vi "Write TDMS.vi"(0 "Queue In":refnum<queue>, 1 "TDMS File In":refnum<k34>, 2 "TDMS Group Names":T3, 3 "Elements Remaning":u32[](array[numeric]), 4 "Logging Channel Cluster":T2, 5 "FIFO Cluster":T1) -> (14 "Logging Channel Cluster":T3, 15 "TDMS Out":refnum<k34>, 16 "Elements Remaining Out":u32[](array[numeric]), 17 "Logging Channel Cluster":T2)   [LabVIEW 2017]
uses:
  Message Queue/Message Cluster.ctl
  Controls/Logging names.ctl
  Message Queue/Message Queue.lvlib
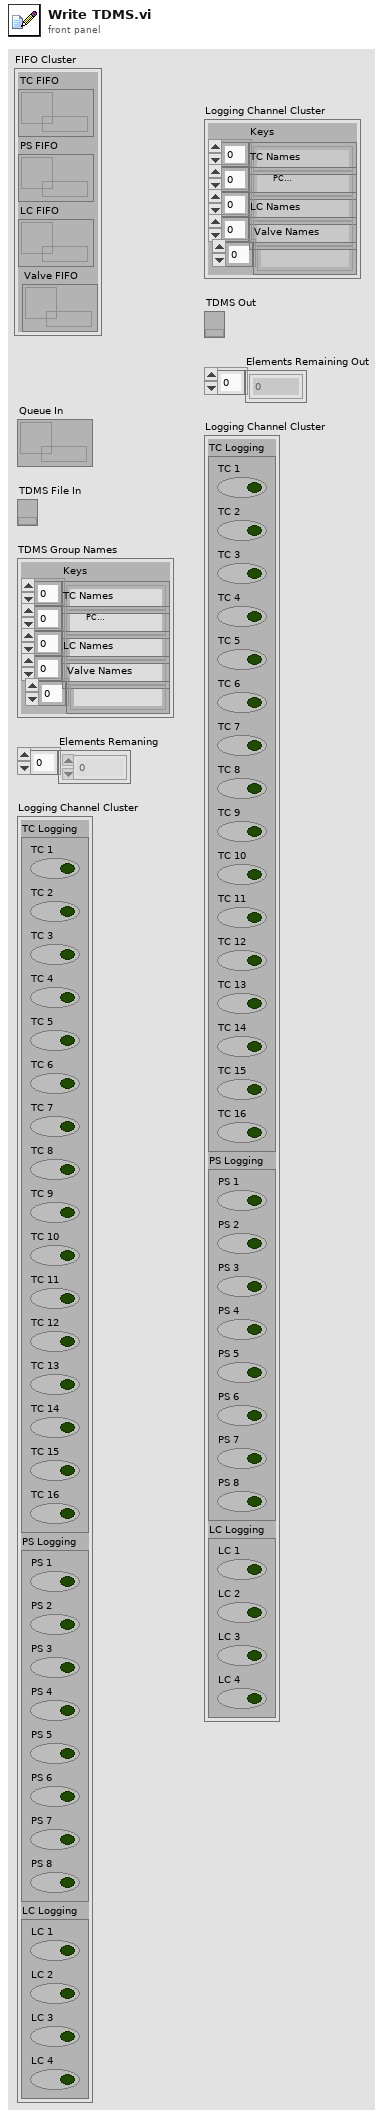
[diagram p1: front panel]
types:
  T1 = cluster{"TC FIFO":refnum<k33>, "PS FIFO":refnum<k33>, "LC FIFO":refnum<k33>, "Valve FIFO":refnum<k33>}
  T2 = cluster{"TC Logging":cluster{"TC 1":bool, "TC 2":bool, "TC 3":bool, "TC 4":bool, "TC 5":bool, "TC 6":bool, "TC 7":bool, "TC 8":bool, "TC 9":bool, "TC 10":bool, "TC 11":bool, "TC 12":bool, "TC 13":bool, "TC 14":bool, "TC 15":bool, "TC 16":bool}, "PS Logging":cluster{"PS 1":bool, "PS 2":bool, "PS 3":bool, "PS 4":bool, "PS 5":bool, "PS 6":bool, "PS 7":bool, "PS 8":bool}, "LC Logging":cluster{"LC 1":bool, "LC 2":bool, "LC 3":bool, "LC 4":bool}}
  T3 = typedef "Logging names.ctl" = cluster{"Keys":string[], "TC Names":string[], "PC Names":string[], "LC Names":string[], "Valve Names":string[]}
  T4 = cluster{"TC 1":bool, "TC 2":bool, "TC 3":bool, "TC 4":bool, "TC 5":bool, "TC 6":bool, "TC 7":bool, "TC 8":bool, "TC 9":bool, "TC 10":bool, "TC 11":bool, "TC 12":bool, "TC 13":bool, "TC 14":bool, "TC 15":bool, "TC 16":bool}
  T5 = cluster{"PS 1":bool, "PS 2":bool, "PS 3":bool, "PS 4":bool, "PS 5":bool, "PS 6":bool, "PS 7":bool, "PS 8":bool}
  T6 = cluster{"LC 1":bool, "LC 2":bool, "LC 3":bool, "LC 4":bool}
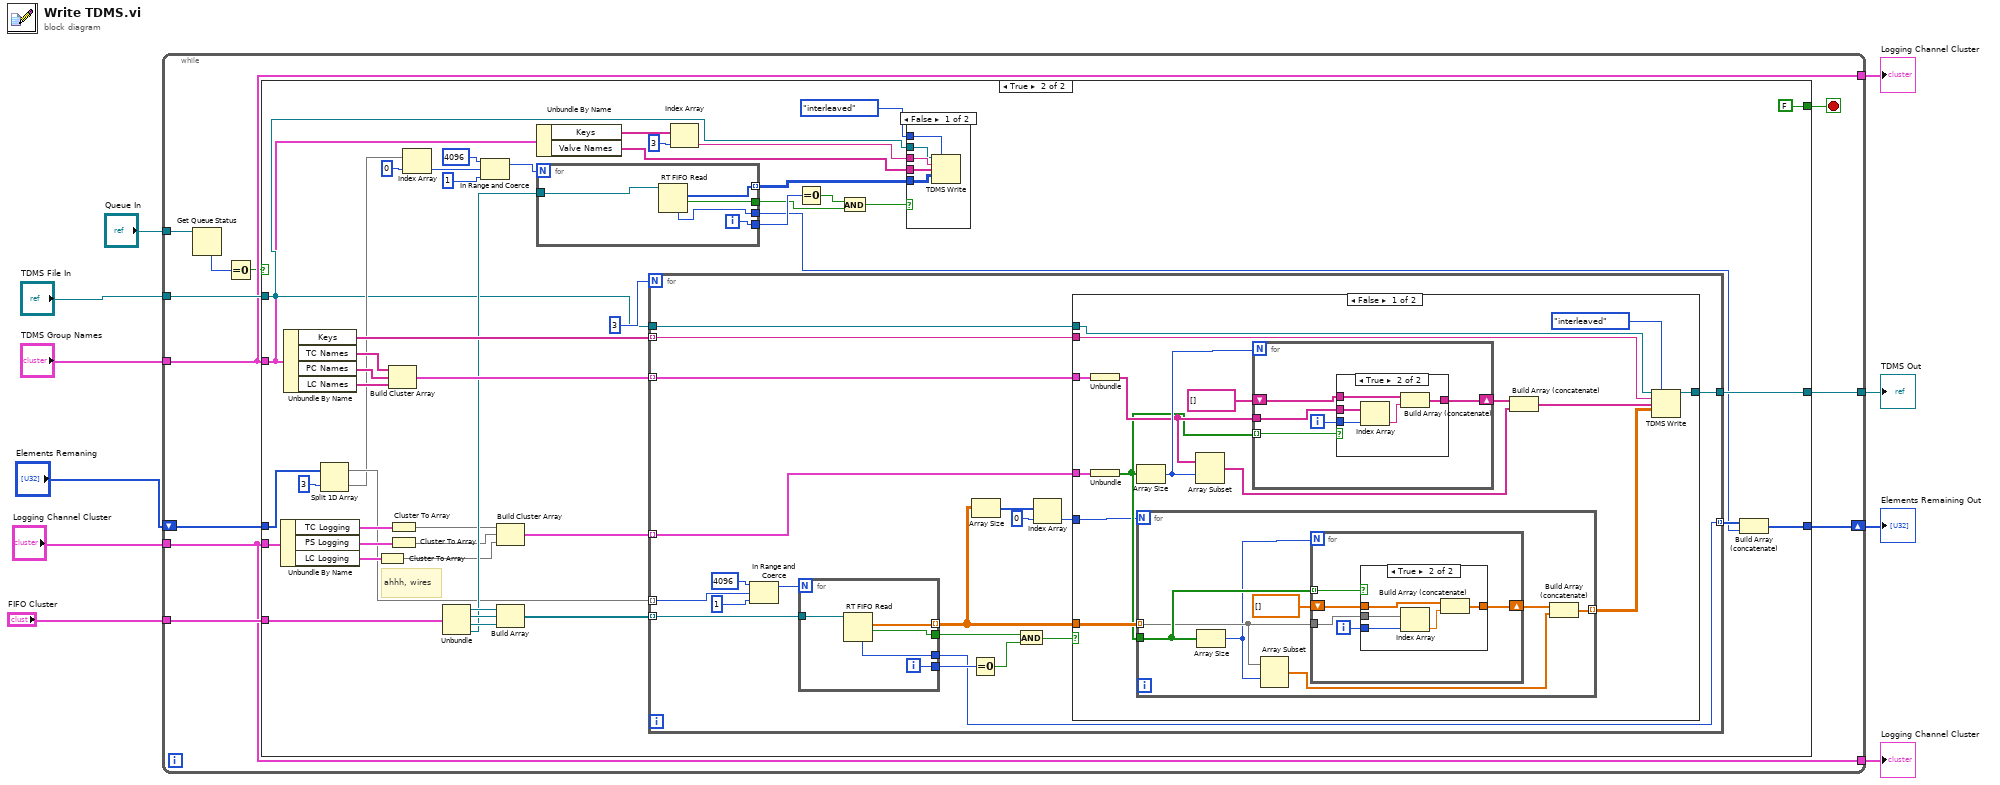
[diagram p0: block diagram]
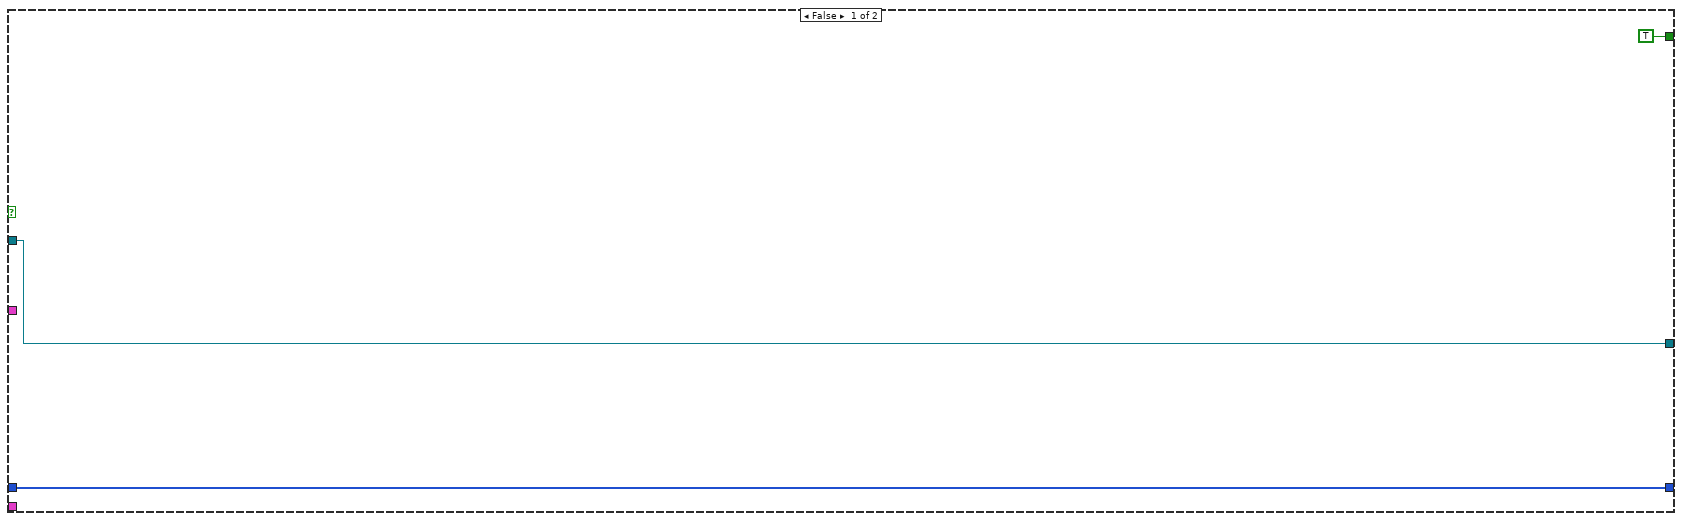
[diagram p2: hidden frame]
diagram:
  n1 = while {
    tunnel: "FIFO Cluster" -> [w17]
    tunnel: [w21] -> w2
    tunnel: "Logging Channel Cluster" -> [w15]
    tunnel: "TDMS Group Names" -> [w16]
    tunnel: "TDMS File In" -> [w18]
    shift-right: [w19] -> w5
    shift-left: "Elements Remaning" -> [w20]
    tunnel: [w15] -> w9
    tunnel: [w16] -> w8
    tunnel: "Queue In" -> [w14]
    stop <- w11 stop-if-true
    n2 = Get Queue Status(queue=w14) -> (# elements in queue=w12:i32)  [unwired: 2 in, 7 out]
    n3 = Equal To 0?(x=w12) -> (x = 0?=w13:bool)
    n4 = case shown="True" w13 {
      tunnel: [w22 w54] -> w21
      tunnel: w20 -> [w23 w41]
      tunnel: [w23 w36] -> w19
      tunnel: w18 -> [w22 w29]
      tunnel: w17 -> [_ w28]
      tunnel: w16 -> [_ w27]
      tunnel: w15 -> [_ w26]
      tunnel: [TRUE FALSE] -> w11
      frame False {
      }
      frame True {
        # "ahhh, wires"
        n5 = Unbundle By Name(w26) -> ("TC Logging"=w53:T4, "PS Logging"=w52:T5, "LC Logging"=w51:T6)
        n6 = Unbundle By Name(w27) -> ("Keys"=w61:string[], "TC Names"=w70:string[], "PC Names"=w69:string[], "LC Names"=w68:string[])
        n7 = Split 1D Array(array=w41, index=3) -> (first subarray=w39:u32[], second subarray=w38:u32[])
        n8 = Cluster To Array(cluster=w51) -> (array=w48:bool[])
        n9 = Build Cluster Array(w70, w69, w68) -> (w62:cluster{"LC Names":string[]}[])
        n10 = Cluster To Array(cluster=w53) -> (array=w50:bool[])
        n11 = Cluster To Array(cluster=w52) -> (array=w49:bool[])
        n12 = Index Array(array=w38, index=0) -> (element=w32:u32)
        n13 = Unbundle(w28) -> ("TC FIFO"=w64:refnum<k33>, "PS FIFO"=w65:refnum<k33>, "LC FIFO"=w66:refnum<k33>, "Valve FIFO"=w60:refnum<k33>)
        n14 = In Range and Coerce(upper limit=u32 4096, x=w32, lower limit=u32 1) -> (coerced(x)=w33:u32)  [unwired: 1 out]
        n15 = Build Cluster Array(w50, w49, w48) -> (w47:cluster{"LC Logging":bool[]}[])
        n16 = Build Array(w64, w65, w66) -> (w63:refnum<k33>[])
        n17 = Unbundle By Name(w27) -> ("Keys"=w59:string[], "Valve Names"=w56:string[])
        n18 = for {
          N: w33 -> [_]
          tunnel: [w74] -> w46 mode=indexing
          tunnel: w60 -> [w75]
          tunnel: [w73] -> w44
          tunnel: [w72] -> w42
          tunnel: [w71] -> w30
          i -> [w73]
          n19 = RT FIFO Read(0:w75) -> (7:w71:u32, 9:w74:i32[], 10:w72:bool)  [unwired: 3 in, 2 out]
        }
        n20 = for {
          N: 3 -> [_]
          tunnel: w63 -> [w99] mode=indexing
          tunnel: w62 -> [w95] mode=indexing
          tunnel: w61 -> [w98] mode=indexing
          tunnel: [w97] -> w54
          tunnel: w47 -> [w94] mode=indexing
          tunnel: w39 -> [w82] mode=indexing
          tunnel: [w86] -> w37 mode=indexing
          tunnel: w29 -> [w81]
          n21 = In Range and Coerce(upper limit=u32 4096, x=w82, lower limit=u32 1) -> (coerced(x)=w83:u32)  [unwired: 1 out]
          n22 = for {
            N: w83 -> [_]
            tunnel: w99 -> [w104]
            tunnel: [w103] -> w96 mode=indexing
            tunnel: [w102] -> w90
            tunnel: [w101] -> w87
            tunnel: [w100] -> w86
            i -> [w102]
            n23 = RT FIFO Read(0:w104) -> (7:w100:u32, 9:w103:sgl[], 10:w101:bool)  [unwired: 3 in, 2 out]
          }
          n24 = Equal To 0?(x=w90) -> (x = 0?=w89:bool)
          n25 = Array Size(array=w96) -> (size(s)=w91:i32[])
          n26 = And(x=w87, y=w89) -> (x .and. y?=w88:bool)
          n27 = Index Array(array=w91, index=0) -> (element=w92:i32)
          n28 = case shown="False" w88 {
            tunnel: w98 -> [w120 _]
            tunnel: [w118 w150] -> w97
            tunnel: w96 -> [w116 _]
            tunnel: w95 -> [w111 _]
            tunnel: w94 -> [w109 _]
            tunnel: w92 -> [w106 _]
            tunnel: w81 -> [w105 w150]
            frame False {
              n29 = Unbundle(w111) -> ("LC Names"=w110:string[])
              n30 = Unbundle(w109) -> ("LC Logging"=w108:bool[])
              n31 = Array Size(array=w108) -> (size(s)=w113:i32)
              n32 = for {
                N: w106 -> [_]
                tunnel: w116 -> [w125] mode=indexing
                tunnel: w108 -> [w127]
                tunnel: [w121] -> w107 mode=indexing
                n33 = Array Size(array=w127) -> (size(s)=w124:i32)
                n34 = Array Subset(array=w125, index=w124) -> (w122:sgl[])  [unwired: 1 in]
                n35 = for {
                  N: w124 -> [_]
                  tunnel: w127 -> [w131] mode=indexing
                  tunnel: w125 -> [w130]
                  shift-right: [w129] -> w123
                  shift-left: sgl[] [] -> [w128]
                  i -> [w132]
                  n36 = case shown="True" w131 {
                    tunnel: w132 -> [_ w138]
                    tunnel: w130 -> [_ w135]
                    tunnel: [w133 w137] -> w129
                    tunnel: w128 -> [w133 w134]
                    frame False {
                    }
                    frame True {
                      n37 = Index Array(array=w135, index=w138) -> (element=w136:sgl)
                      n38 = Build Array (concatenate)(w134, w136) -> (w137:sgl[])
                    }
                  }
                }
                n39 = Build Array (concatenate)(w123, w122) -> (w121:sgl[])
              }
              n40 = Array Subset(array=w110, index=w113) -> (w112:string[])  [unwired: 1 in]
              n41 = for {
                N: w113 -> [_]
                tunnel: w108 -> [w143] mode=indexing
                tunnel: w110 -> [w141]
                shift-right: [w139] -> w114
                shift-left: string[] [] -> [w140]
                i -> [w142]
                n42 = case shown="True" w143 {
                  tunnel: w142 -> [_ w148]
                  tunnel: w141 -> [_ w149]
                  tunnel: w140 -> [w144 w146]
                  tunnel: [w144 w145] -> w139
                  frame False {
                  }
                  frame True {
                    n43 = Index Array(array=w149, index=w148) -> (element=w147:string)
                    n44 = Build Array (concatenate)(w146, w147) -> (w145:string[])
                  }
                }
              }
              n45 = Build Array (concatenate)(w114, w112) -> (w117:string[])
              n46 = TDMS Write(0:w105, 1:enum16{"decimated", "interleaved"}."interleaved" ("data layout (0:decimated)"), 5:w120, 7:w117, 9:w107) -> (4:w118:refnum<k34>)  [unwired: 1 in, 3 out]
            }
            frame True {
            }
          }
        }
        n47 = Index Array(array=w59, index=3) -> (element=w57:string)
        n48 = Equal To 0?(x=w44) -> (x = 0?=w45:bool)
        n49 = And(x=w45, y=w42) -> (x .and. y?=w43:bool)
        n50 = case shown="False" w43 {
          tunnel: w46 -> [w80 _]
          tunnel: w57 -> [w79 _]
          tunnel: w29 -> [w78 _]
          tunnel: w56 -> [w77 _]
          tunnel: enum16{"decimated", "interleaved"}."interleaved" ("data layout (0:decimated)") -> [w76 _]
          frame False {
            n51 = TDMS Write(0:w78, 1:w76, 5:w79, 7:w77, 9:w80) -> ()  [unwired: 1 in, 4 out]
          }
          frame True {
          }
        }
        n52 = Build Array (concatenate)(w37, w30) -> (w36:u32[])
      }
    }
  }
  "Logging Channel Cluster" <- w9
  "Logging Channel Cluster" <- w8
  "Elements Remaining Out" <- w5
  "TDMS Out" <- w2
